vi "Set Column Values.vi"(7 "Sheet Name":string, 8 "error in":errorcluster, 9 "Values":variant[](array[variant]), 10 "Cell Address":string, 11 "SpreadsheetDoc":refnum<k24>) -> (0 "error out":errorcluster, 3 "SpreadsheetDoc out":refnum<k24>)   [LabVIEW 2019, in "Open Xml.lvlib"]
uses:
  Open Xml.lvlib
  D:/git/Open-Xml-LabVIEW/Source/DocumentFormat.OpenXml.dll
  DocumentFormat.OpenXml.dll
  9d8afaec-d2fb-40ec-934f-6b6fb5d78b9a.vi
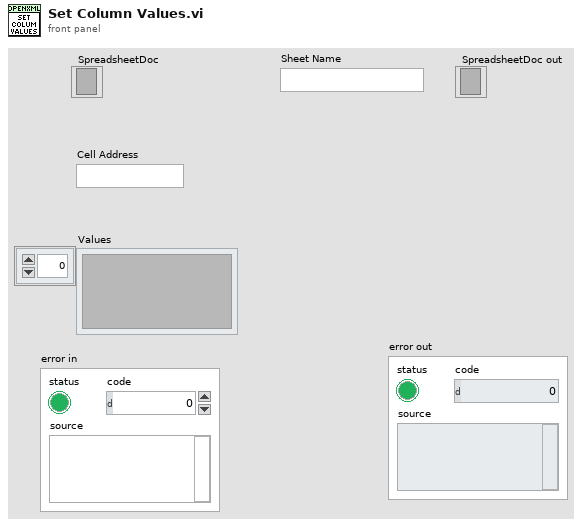
[diagram p1: front panel]
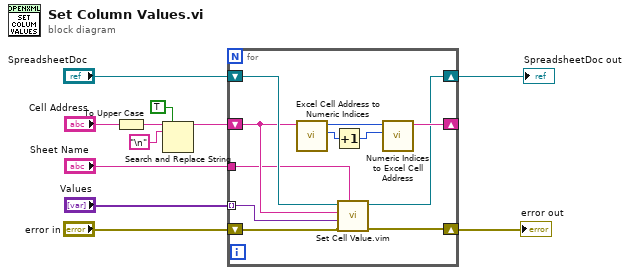
[diagram p0: block diagram]
diagram:
  n1 = To Upper Case(1:"Cell Address") -> (0:w6:string)
  n2 = Search and Replace String(replace all?=TRUE ("replace all? (F)"), input string=w6, search string="\n") -> (result string=w5:string)  [unwired: 5 in, 3 out]
  n3 = for {
    tunnel: "Values" -> [w14] mode=indexing
    shift-right: [w13] -> w3
    shift-left: "error in" -> [w18]
    shift-right: [w21] -> _
    shift-left: w5 -> [w16]
    shift-right: [w15] -> w2
    shift-left: "SpreadsheetDoc" -> [w17]
    tunnel: "Sheet Name" -> [w12]
    n4 = call "Excel Cell Address to Numeric Indices.vi"("Cell Name"=w16) -> ("Row Number"=w22:i32, "Column Number"=w20:i32)  [unwired: 9 in]
    n5 = Increment(x=w22) -> (x+1=w19:i32)
    n6 = call "Set Cell Value.vim"("Sheet Name"=w12, "error in"=w18, "Value"=w14, "Cell Address"=w16, "SpreadsheetDoc in"=w17) -> ("error out"=w13:errorcluster, "SpreadsheetDoc out"=w15:refnum<k24>)  [unwired: 5 in]
    n7 = call "Numeric Indices to Excel Cell Address.vi"("Row"=w19, "Column"=w20) -> ("Cell Address"=w21:string)  [unwired: 9 in]
  }
  "SpreadsheetDoc out" <- w2
  "error out" <- w3
